vi "Get Terminal by ID.vi"(8 "error in (no error)":errorcluster, 10 "ID":i32, 11 "Data Cluster in":T1) -> (0 "error out":errorcluster, 2 "specific class reference":refnum<vi>, 3 "Data Cluster out":T1)   [LabVIEW 2025, in "Scripting Server.lvlib"]
uses:
  Scripting Server.lvlib
  Module Data--cluster.ctl
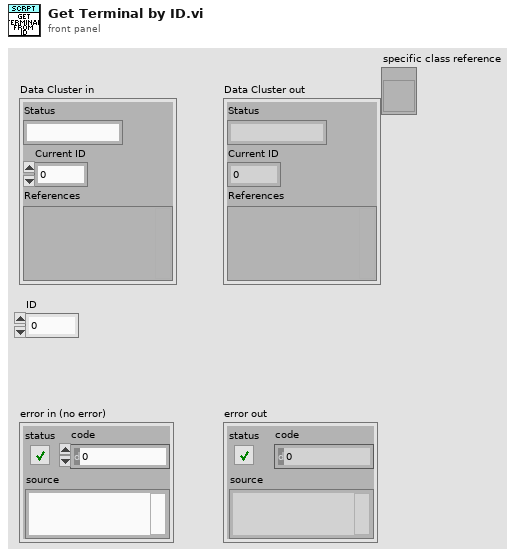
[diagram p1: front panel]
types:
  T1 = typedef "Scripting Server.lvlib/Module Data--cluster.ctl" = cluster{"Status":string, "Current ID":i32, "References":variant}
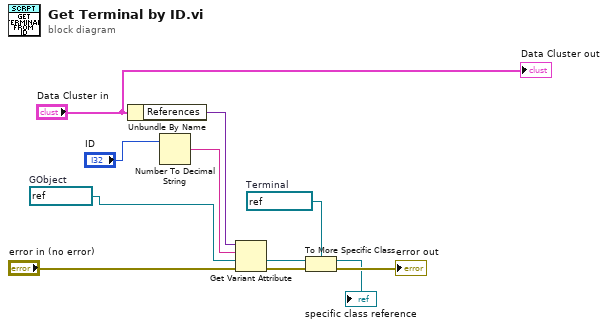
[diagram p0: block diagram]
diagram:
  w2 = refnum<vi> refnum  # Terminal
  w5 = refnum<vi> refnum  # GObject
  n1 = Unbundle By Name("Data Cluster in") -> ("References"=w9:variant)
  n2 = Number To Decimal String(number="ID") -> (decimal integer string=w10:string)  [unwired: 1 in]
  n3 = Get Variant Attribute(Variant=w9, name=w10, default value (empty Variant)=w5, error in="error in (no error)") -> (value=w3:refnum<vi>, error out=w11:errorcluster)  [unwired: 2 out]
  n4 = To More Specific Class(target class=w2, reference=w3, error in=w11) -> (specific class reference=→"specific class reference":refnum<vi>, error out=→"error out":errorcluster)
  "Data Cluster out" <- "Data Cluster in"
